vi "libssh2_userauth_publickey_fromfile_ex.vi"(5 "private key":path, 7 "public key":path, 8 "error in (no error)":errorcluster, 9 "passphrase":string, 10 "username":string, 11 "session":T1) -> (0 "error out":errorcluster)   [LabVIEW 2013, in "libssh2.lvlib"]
doc: "Authenticate a session using a private and public key file."
uses:
  libssh2.lvlib
  Session Refnum.ctl
  Not A Session.vi
  <vilib>/Utility/error.llb/Error Cluster From Error Code.vi
  Global Settings.vi
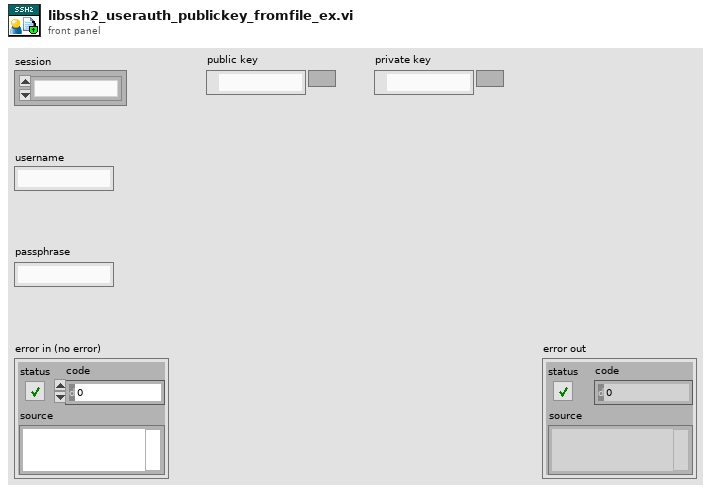
[diagram p1: front panel]
types:
  T1 = typedef "libssh2.lvlib/Session Refnum.ctl" = refnum<k1>
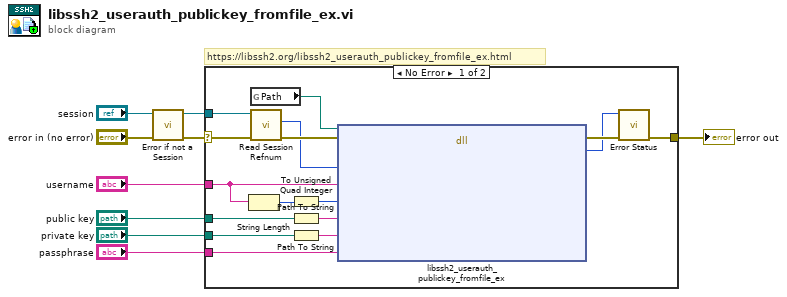
[diagram p0: block diagram]
diagram:
  # "https://libssh2.org/libssh2_userauth_publickey_fromfile_ex.html"
  n1 = call "Error if not a Session.vi"("error in (no error)"="error in (no error)", "session"="session") -> ("error out"=w6:errorcluster, "session out"=w4:T1)  [unwired: 8 in]
  n2 = case shown="No Error" w6 {
    selector: w6 -> [w24 w26]
    tunnel: "username" -> [w25 _]
    tunnel: [w23 w26] -> w8
    tunnel: w4 -> [w22 _]
    tunnel: "public key" -> [w14 _]
    tunnel: "private key" -> [w13 _]
    tunnel: "passphrase" -> [w12 _]
    frame No Error {
      n3 = String Length(string=w25) -> (length=w19:i32)
      n4 = global read "Global Settings.vi" "Path"() -> (w16:path)
      n5 = call "Read Session Refnum.vi"("error in (no error)"=w24, "session"=w22) -> ("error out"=w18:errorcluster, "LIBSSH2_SESSION*"=w17:u64)  [unwired: 5 in, 3 out]
      n6 = To Unsigned Quad Integer(1:w19) -> (0:w21:u64)
      n7 = Path To String(path=w14) -> (string=w11:string)
      n8 = Path To String(path=w13) -> (string=w10:string)
      n9 = dll-call lib="?" fn="libssh2_userauth_publickey_fromfile_ex"(path in=w16, error in=w18, "session"=w17, "username"=w25, "username_len"=w21, "publickey"=w11, "privatekey"=w10, "passphrase"=w12) -> (error out=w20:errorcluster, "return value"=w15:i32)  [unwired: 7 in, 1 out]
      n10 = call "Error Status.vi"("error in (no error)"=w20, "return value"=w15) -> ("error out"=w23:errorcluster)  [unwired: 8 in, 1 out]
    }
    frame Error {
    }
  }
  "error out" <- w8
